vi "PathSup2Lines.vi"(8 "ColorMap":T1=52 items=["Bathymetry9", "BlackBody", "Blue", "BlueBlackRed", "BlueGreenOrange", "BlueHot", "BlueHot256", "BlueRedGreen", "BlueRedGreen256", "BrownViolet", "Classification", "ColdWarm", "Copper", "Cyan", "CyanMagenta", "Cycles", "dBZ14", "dBZ21", "EOSOrangeBlue11", "EOSSpectral11", "Fiddle", "Geo", "Geo32", "Gold", "Grays", "Grays16", "Grays256", "Green", "GreenMagenta16", "LandAndSea", "LandAndSea8", "Magenta", "Mocha", "Mud", "Pastels", "PastelsMap", "PastelsMap20", "PlanetEarth", "PlanetEarth256", "Rainbow", "Rainbow4Cycles", "Rainbow16", "Rainbow256", "RainbowCycle", "Red", "RedWhiteBlue", "RedWhiteBlue256", "RedWhiteGreen", "Relief", "Relief19", "SeaLandAndFire", "Spectrum", "SpectrumBlack", "Terrain", "Terrain256", "VioletOrangeYellow", "Web216", "Yellow", "YellowHot", "YellowHot256"], 9 "HighPower":dbl=1.0, 10 "Z":dbl format="%#_13g", 11 "PathSupreme":T3) -> (2 "Colors":u32[](array[numeric]), 3 "Lines":cluster{"P0":T2, "P1":T2}[](array[cluster]))   [LabVIEW 2014]
uses:
  TypeDefs/PathSupreme.ctl
  PSup2SCAN/Sub/VelocityProfile.ctl
  PSup2SCAN/Sub/PathCut.ctl
  PSup2SCAN/Sub/Segment.ctl
  TypeDefs/Point3D.ctl
  ColorMaps.ctl
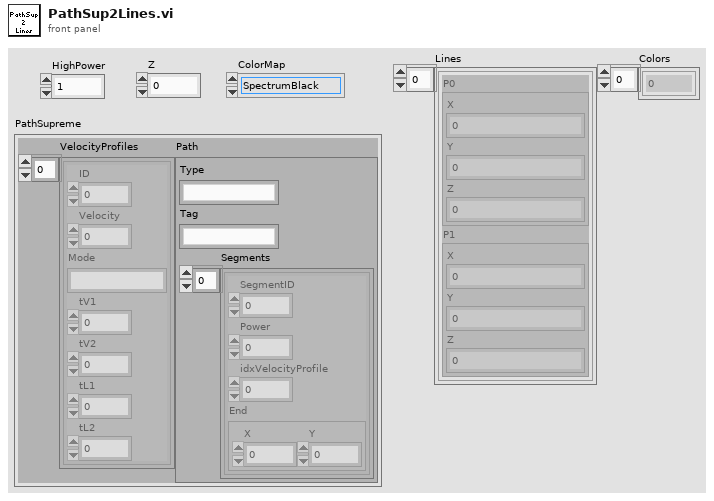
[diagram p1: front panel]
types:
  T1 = typedef "ColorMaps.ctl" = u16
  T2 = typedef "Point3D.ctl" = cluster{"X":sgl, "Y":sgl, "Z":sgl}
  T3 = typedef "PathSupreme.ctl" = cluster{"VelocityProfiles":T4[], "Path":T5}
  T4 = typedef "VelocityProfile.ctl" = cluster{"ID":u32, "Velocity":dbl, "Mode":string, "tV1":u32, "tV2":u32, "tL1":u32, "tL2":u32}
  T5 = typedef "PathCut.ctl" = cluster{"Type":string, "Tag":string, "Segments":T6[]}
  T6 = typedef "Segment.ctl" = cluster{"SegmentID":u16, "Power":sgl, "idxVelocityProfile":u16, "End":cluster{"X":sgl, "Y":sgl}}
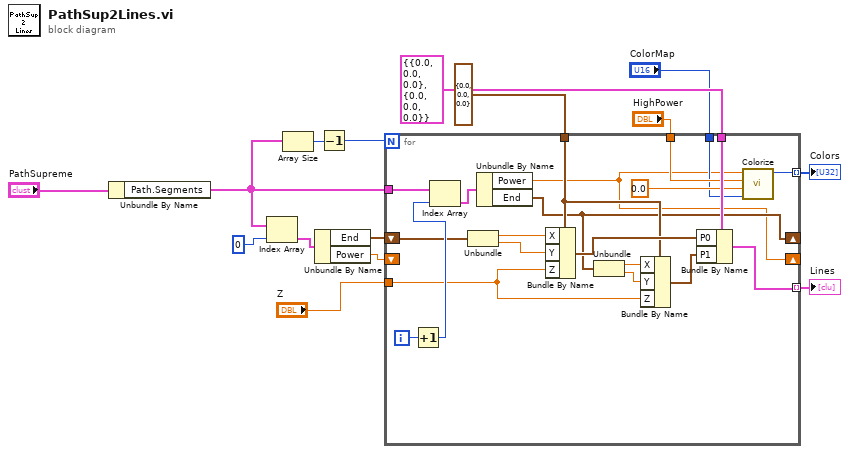
[diagram p0: block diagram]
diagram:
  n1 = Unbundle By Name("PathSupreme") -> ("Path.Segments"=w12:T6[])
  n2 = Index Array(array=w12, index=0) -> (element=w10:T6)
  n3 = Array Size(array=w12) -> (size(s)=w14:i32)
  n4 = Unbundle By Name(w10) -> ("End"=w9:cluster{"X":sgl, "Y":sgl}, "Power"=w1:sgl)
  n5 = Decrement(x=w14) -> (x-1=w13:i32)
  n6 = for {
    N: w13 -> [_]
    tunnel: w12 -> [w36]
    shift-right: [w22] -> _
    shift-left: w9 -> [w31]
    tunnel: cluster{"P0":T2, "P1":T2} {"P0"={"X"=0.0, "Y"=0.0, "Z"=0.0}, "P1"={"X"=0.0, "Y"=0.0, "Z"=0.0}} ("Line") -> [w32]
    tunnel: T2 {"X"=0.0, "Y"=0.0, "Z"=0.0} ("P0") -> [w27]
    tunnel: "Z" -> [w24]
    tunnel: [w21] -> w5 mode=indexing
    tunnel: "HighPower" -> [w20]
    tunnel: "ColorMap" -> [w18]
    tunnel: [w17] -> w2 mode=indexing
    shift-right: [w16] -> _
    shift-left: w1 -> [_]
    i -> [w35]
    n7 = Increment(x=w35) -> (x+1=w34:i32)
    n8 = Index Array(array=w36, index=w34) -> (element=w33:T6)
    n9 = Unbundle(w31) -> ("X"=w30:sgl, "Y"=w29:sgl)
    n10 = Unbundle By Name(w33) -> ("Power"=w16:sgl, "End"=w22:cluster{"X":sgl, "Y":sgl})
    n11 = Bundle By Name(cluster=w27, "X"=w30, "Y"=w29, "Z"=w24) -> (w28:T2)
    n12 = Unbundle(w22) -> ("X"=w26:sgl, "Y"=w25:sgl)
    n13 = Bundle By Name(cluster=w27, "X"=w26, "Y"=w25, "Z"=w24) -> (w23:T2)
    n14 = Bundle By Name(cluster=w32, "P0"=w28, "P1"=w23) -> (w21:cluster{"P0":T2, "P1":T2})
    n15 = call "Colorize.vi"("ColorMap"=w18, "Low"=0.0, "High"=w20, "ValueIn"=w16) -> ("ColorOut"=w17:u32)  [unwired: 7 in]
  }
  "Lines" <- w5
  "Colors" <- w2
